vi "cook.vi"(8 "error in (no error)":errorcluster, 11 "Pop in":refnum<class "Pop.lvclass">) -> (0 "error out":errorcluster, 3 "Pop out":refnum<class "Pop.lvclass">)   [LabVIEW 2010, in "CookBehaviors.lvlib" / "Pop.lvclass"]
uses:
  Pop.lvclass
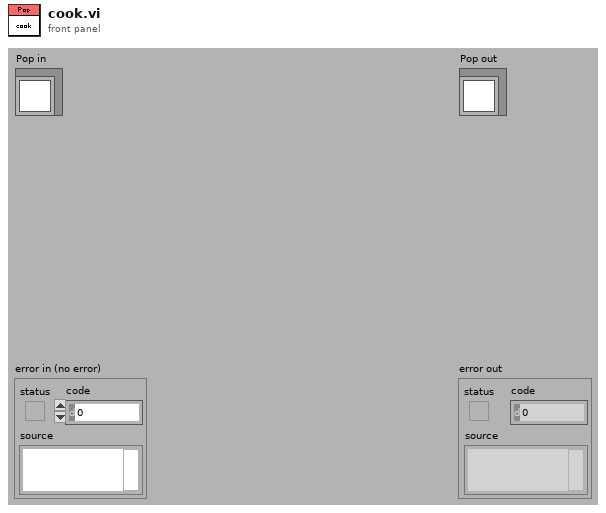
[diagram p1: front panel]
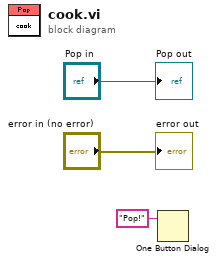
[diagram p0: block diagram]
diagram:
  n1 = One Button Dialog(message="Pop!") -> ()  [unwired: 1 in, 1 out]
  "error out" <- "error in (no error)"
  "Pop out" <- "Pop in"
